vi "Get Invoke __Input.vi"(8 "error in (no error)":errorcluster, 11 "gRPCid":T2) -> (0 "error out":errorcluster, 2 "Message Data":T1, 3 "gRPCid out":T2)   [LabVIEW 2019, in "OOP Server.lvlib" / "OOP Server.lvclass"]
uses:
  OOP Server.lvclass
  gRPC interface/Server API/typeDefs/grpcId.ctl
  gRPC interface/gprc-lvsupport.lvlib
  RPC Messages/InvokeRequest/InvokeRequest_Data.ctl
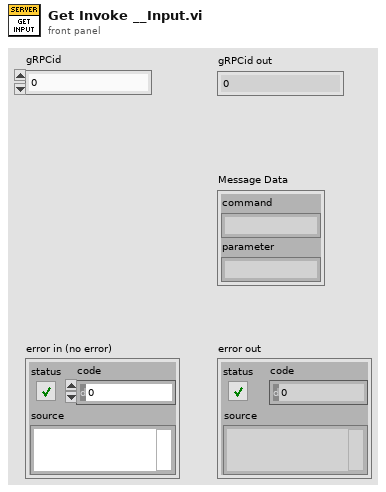
[diagram p1: front panel]
types:
  T1 = typedef "OOP Server.lvlib/OOP Server.lvclass/InvokeRequest_Data.ctl" = cluster{"command":string, "parameter":string}
  T2 = typedef "gprc-lvsupport.lvlib/grpcId.ctl" = u64
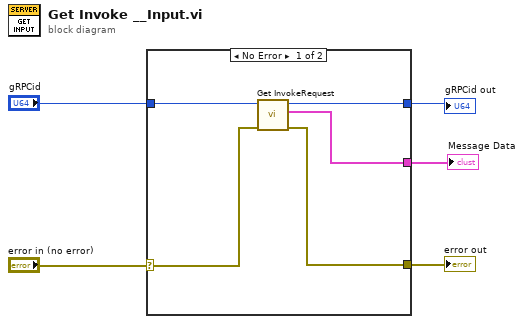
[diagram p0: block diagram]
diagram:
  n1 = case shown="No Error" "error in (no error)" {
    selector: "error in (no error)" -> [w6 w11]
    tunnel: "gRPCid" -> [w10 w12]
    tunnel: [w9 w12] -> w4
    tunnel: [w8 w11] -> w3
    tunnel: [w7 _] -> w2
    frame No Error {
      n2 = call "Get InvokeRequest.vi"("error in (no error)"=w6, "gRPCid"=w10) -> ("error out"=w8:errorcluster, "Request Data"=w7:T1, "gRPCid out"=w9:T2)  [unwired: 7 in]
    }
    frame Error {
    }
  }
  "error out" <- w3
  "gRPCid out" <- w4
  "Message Data" <- w2
